vi "Noise Processing.vi"(8 "Min Voltage":dbl format="%.2f", 9 "Max Voltage":dbl format="%.2f", 10 "16-bit Binary":bool, 11 "Data":dbl[](array[numeric]) format="%.6f") -> (0 "ENOB (RMS)":dbl format="%.2f", 1 "ENOB (max-min)":dbl format="%.2f", 2 "16-bit Binary Results":T1 {"max-min" format="%.9f"; "Min" format="%.9f"; "Max" format="%.9f"; "Std Dev (RMS)" format="%.9f"; "Avg" format="%.9f"}, 3 "Results":T1 {"max-min" format="%.9f"; "Min" format="%.9f"; "Max" format="%.9f"; "Std Dev (RMS)" format="%.9f"; "Avg" format="%.9f"}, 4 "Binary Data":dbl[](array[numeric]) format="%.2f")   [LabVIEW 2024]
uses:
  <vilib>/Analysis/NI_AALBase.lvlib
panel:
  out "log2(SD)":dbl format="%.2g"
  # "Only needed if \"16-bit Binary\" is False."
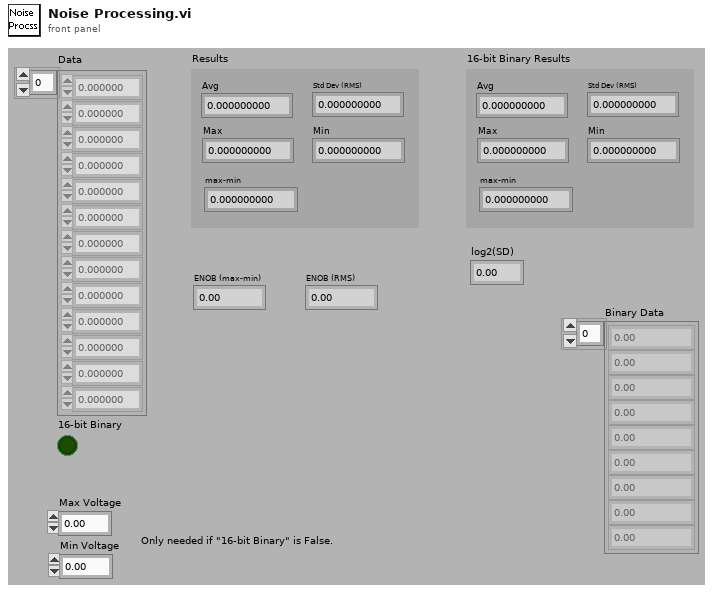
[diagram p1: front panel]
types:
  T1 = cluster{"Avg":dbl, "Std Dev (RMS)":dbl, "Max":dbl, "Min":dbl, "max-min":dbl}
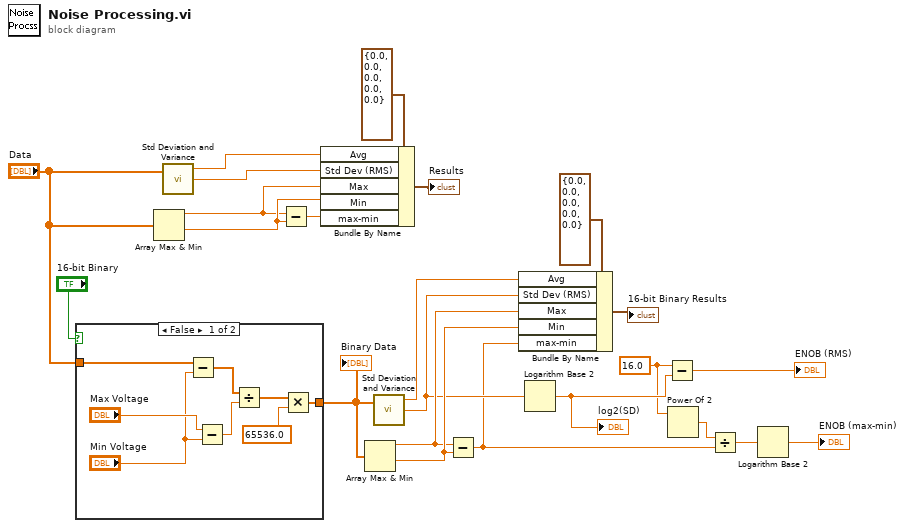
[diagram p0: block diagram]
diagram:
  w18 = 16.0 ("x")
  n1 = case shown="False" "16-bit Binary" {
    tunnel: "Data" -> [w30 w32]
    tunnel: [w24 w32] -> w16
    frame False {
      n2 = Subtract(x=w30, y="Min Voltage") -> (x-y=w28:dbl[])
      n3 = Subtract(x="Max Voltage", y="Min Voltage") -> (x-y=w27:dbl)
      n4 = Divide(x=w28, y=w27) -> (x/y=w26:dbl[])
      n5 = Multiply(x=w26, y=65536.0 ("x")) -> (x*y=w24:dbl[])
    }
    frame True {
    }
  }
  "Binary Data" <- w16
  n6 = Array Max & Min(array="Data") -> (max value=w10:dbl, min value=w11:dbl)  [unwired: 2 out]
  n7 = call <vilib>:"Std Deviation and Variance.vi"("X"="Data") -> ("mean"=w8:dbl, "standard deviation"=w9:dbl)  [unwired: 1 in, 1 out]
  n8 = Subtract(x=w10, y=w11) -> (x-y=w12:dbl)
  n9 = Bundle By Name(cluster=T1 {"Avg"=0.0, "Std Dev (RMS)"=0.0, "Max"=0.0, "Min"=0.0, "max-min"=0.0} ("Results"), "Avg"=w8, "Std Dev (RMS)"=w9, "Max"=w10, "Min"=w11, "max-min"=w12) -> (→"Results":T1)
  n10 = Array Max & Min(array=w16) -> (max value=w4:dbl, min value=w5:dbl)  [unwired: 2 out]
  n11 = call <vilib>:"Std Deviation and Variance.vi"("X"=w16) -> ("mean"=w2:dbl, "standard deviation"=w3:dbl)  [unwired: 1 in, 1 out]
  n12 = Subtract(x=w4, y=w5) -> (x-y=w1:dbl)
  n13 = Bundle By Name(cluster=T1 {"Avg"=0.0, "Std Dev (RMS)"=0.0, "Max"=0.0, "Min"=0.0, "max-min"=0.0} ("Results"), "Avg"=w2, "Std Dev (RMS)"=w3, "Max"=w4, "Min"=w5, "max-min"=w1) -> (→"16-bit Binary Results":T1)
  n14 = Logarithm Base 2(1:w3) -> (0:w20:dbl)
  "log2(SD)" <- w20
  n15 = Subtract(x=w18, y=w20) -> (x-y=→"ENOB (RMS)":dbl)
  n16 = Power Of 2(x=w18) -> (2^x=w21:dbl)
  n17 = Divide(x=w21, y=w1) -> (x/y=w22:dbl)
  n18 = Logarithm Base 2(1:w22) -> (0:→"ENOB (max-min)":dbl)
